vi "testNoError.vi"() -> ()   [LabVIEW 2017, in "Assertion.Tests.lvlib" / "AssertNoError.lvlib"]
uses:
  AssertNoError.lvlib
  Assertion/Assertion.lvlib
panel:
  out "error out":errorcluster
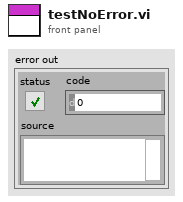
[diagram p1: front panel]
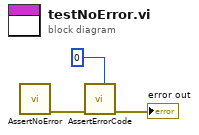
[diagram p0: block diagram]
diagram:
  n1 = call "AssertNoError.vi"() -> ("error out"=w1:errorcluster)  [unwired: 11 in]
  n2 = call "AssertErrorCode.vi"("Expected"=0, "error in (no error)"=w1) -> ("error out"=→"error out":errorcluster)  [unwired: 9 in]
